vi "Starting.vi"(4 "Queue of Async Elements":refnum<queue>, 6 "Actor Ref":refnum<vi>, 7 "Actor in":refnum<class "Actor.lvclass">, 9 "Attributes":refnum<class "Attributes.lvclass">, 10 "Refs":refnum<class "Refs.lvclass">) -> (0 "Error out":errorcluster, 5 "Actor out":refnum<class "Actor.lvclass">)   [LabVIEW 2025, in "jettl.lvlib" / "Notifier Transport.lvlib"]
uses:
  Notifier Transport.lvlib
  jettl.lvlib
  Actor/Actor.lvclass
  Attributes/Attributes.lvclass
  Refs/Refs.lvclass
  Async Elements.ctl
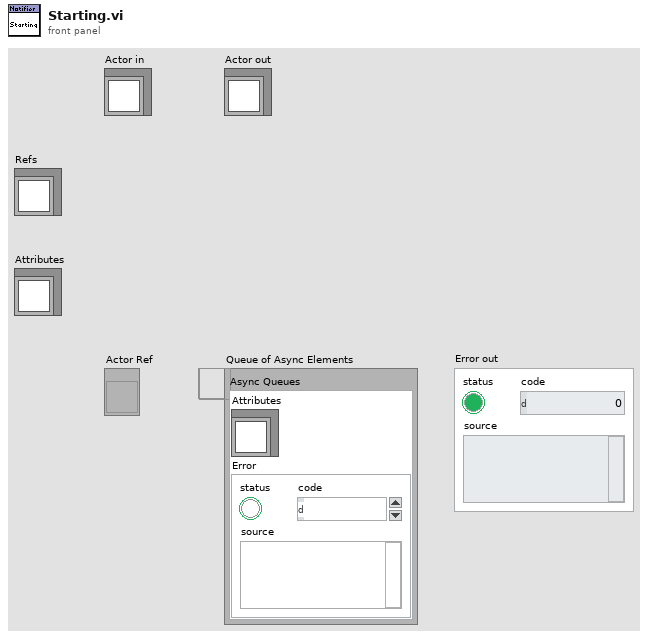
[diagram p1: front panel]
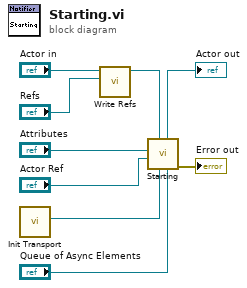
[diagram p0: block diagram]
diagram:
  n1 = call "Init Transport.vi"() -> ("Transport"=w2:refnum<class "Transport.lvclass">)  [unwired: 11 in]
  n2 = call-dynamic "Write Refs.vi"("Refs"="Refs", "Actor in"="Actor in") -> ("Actor out"=w5:refnum<class "Actor.lvclass">)  [unwired: 9 in]
  n3 = call "Starting.vi"("Queue of Async Elements"="Queue of Async Elements", "Transport"=w2, "Actor in"=w5, "Actor Ref"="Actor Ref", "Attributes"="Attributes") -> ("Error out"=→"Error out":errorcluster, "Actor out"=→"Actor out":refnum<class "Actor.lvclass">)  [unwired: 5 in]
